vi "Load Program From String.vi"(8 "Error In":errorcluster, 10 "OpenCL Source Code":string, 11 "Device In":T2) -> (0 "Error Out":errorcluster, 2 "Program Handle":T1, 3 "Device Out":T2)   [LabVIEW 2012]
doc: "Loads a specified program from a string. If the string is not valid or empty, a GUI is launched to help configure a program.\n\nThe GUI has options to load a program, save a program, compile a program, cancel the GUI, or finish the program. Please see the manual for more details."
uses:
  Non-User VIs/Controls/Device ID.ctl
  Non-User VIs/Controls/Program Handle.ctl
  OpenCLV x64.lvlib
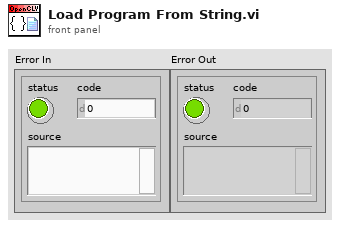
[diagram p1: front panel]
types:
  T1 = typedef "OpenCLV x64.lvlib/Program Handle.ctl" = u64
  T2 = typedef "OpenCLV x64.lvlib/Device ID.ctl" = u64
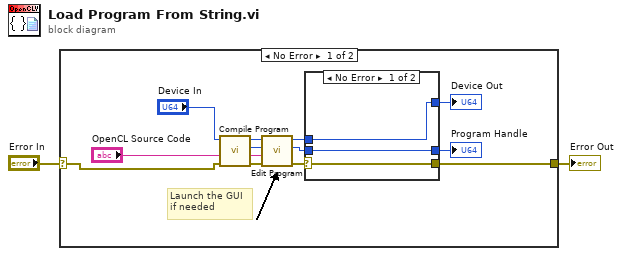
[diagram p0: block diagram]
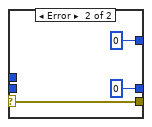
[diagram p2: hidden frame]
diagram:
  n1 = case shown="No Error" "Error In" {
    selector: "Error In" -> [w3 w22]
    tunnel: [w11 w22] -> w1
    frame No Error {
      # "Launch the GUI\nif needed"
      n2 = call "Compile Program.vi"("error in (no error)"=w3, "OpenCL Source Code"="OpenCL Source Code", "Device In in"="Device In") -> ("error out"=w10:errorcluster, "OpenCL Source Code Out"=w7:string, "Program Handle"=w8:T1, "Device Out"=w9:T2)  [unwired: 5 in]
      n3 = call "Edit Program.vi"("Error In"=w10, "Program Source"=w7, "Program Handle"=w8, "Device In"=w9) -> ("Error Out"=w14:errorcluster, "Program Handle"=w13:T1, "Device Out"=w12:T2)  [unwired: 5 in]
      n4 = case shown="No Error" w14 {
        selector: w14 -> [w18 w21]
        tunnel: w12 -> [w17 _]
        tunnel: w13 -> [w16 _]
        tunnel: [w18 w21] -> w11
        tunnel: [w17 T2 0 ("Device Out")] -> w5
        tunnel: [w16 T1 0 ("Program Handle")] -> w4
        frame No Error {
        }
        frame Error {
        }
      }
      "Program Handle" <- w4
      "Device Out" <- w5
    }
    frame Error {
    }
  }
  "Error Out" <- w1
